vi "message box mobile.vi"(11 "String":string="Searching for serial ports...\nPlease wait..") -> ()   [LabVIEW 2016]
uses:
  message box enable.vi
panel:
  out "Gauge":dbl(knob)=58.0 min=0.0 max=100.0 scale=0.0..100.0
  in  "OK Button":bool
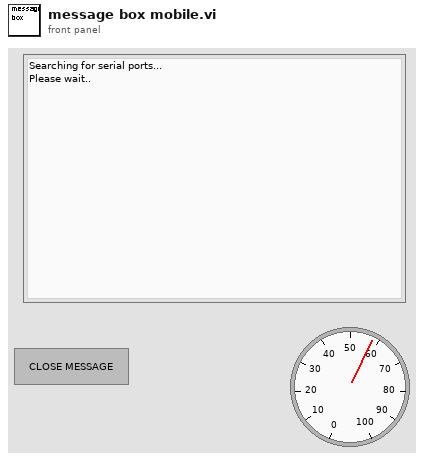
[diagram p1: front panel]
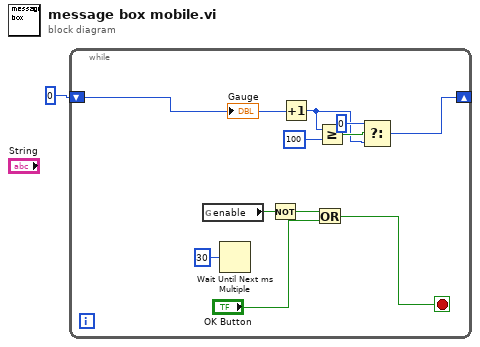
[diagram p0: block diagram]
diagram:
  n1 = while {
    shift-right: [w3] -> _
    shift-left: 0 -> [w7]
    stop <- w8 stop-if-true
    n2 = global read "message box enable.vi" "enable"() -> (w11:bool)
    n3 = Wait Until Next ms Multiple(millisecond multiple=u32 30) -> ()  [unwired: 1 out]
    n4 = Not(x=w11) -> (.not. x?=w10:bool)
    n5 = Increment(x=w7) -> (x+1=w4:i32)
    n6 = Or(x=w10, y="OK Button") -> (x .or. y?=w8:bool)
    n7 = Greater Or Equal?(x=w4, y=100) -> (x >= y?=w6:bool)
    n8 = Select(t=0, s=w6, f=w4) -> (s? t:f=w3:i32)
    "Gauge" <- w7
  }
